vi "Add Device.vi"(8 "error in":errorcluster) -> (0 "error out":errorcluster)   [LabVIEW 2024, in "Data Base.lvlib"]
uses:
  Data Base.lvlib
  Support/General Type Defs/Global Data.vi
  Support/General Type Defs/General Type Defs.lvlib
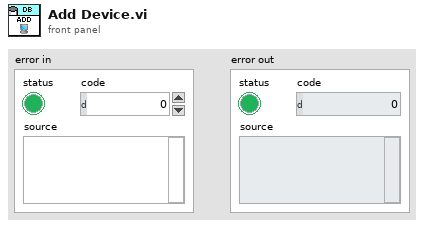
[diagram p1: front panel]
types:
  T1 = typedef "General Type Defs.lvlib/Device Data.ctl" = cluster{"OS":T2, "User":string, "Password":string, "Hostname":string, "IP Address":string}
  T2 = typedef "General Type Defs.lvlib/Device OS.ctl" = enum16{"Windows", "Linux"}
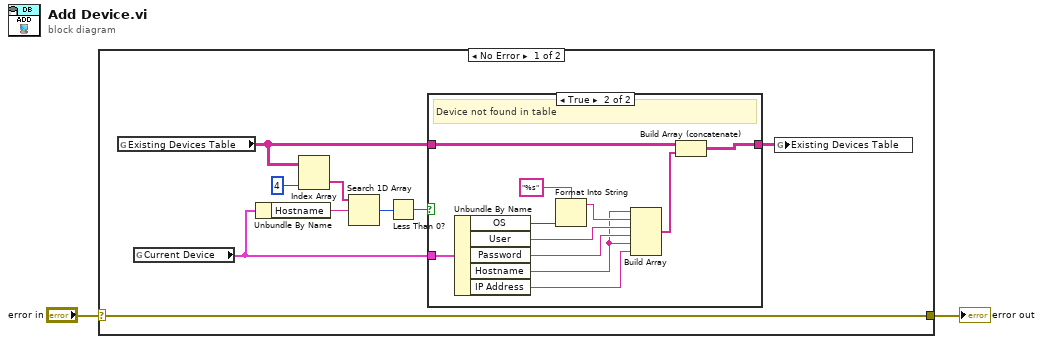
[diagram p0: block diagram]
diagram:
  n1 = case shown="No Error" "error in" {
    selector: "error in" -> [w5 w24]
    tunnel: [w5 w24] -> w1
    frame No Error {
      n2 = global read "Global Data.vi" "Existing Devices Table"() -> (w4:string[][])
      n3 = global read "Global Data.vi" "Current Device"() -> (w11:T1)
      n4 = Unbundle By Name(w11) -> ("Hostname"=w8:string)
      n5 = Index Array(array=w4, index (col)=4) -> (element=w9:string[])  [unwired: 1 in]
      n6 = Search 1D Array(1D array=w9, element=w8) -> (index of element=w7:i32)  [unwired: 1 in]
      n7 = Less Than 0?(x=w7) -> (x < 0?=w6:bool)
      n8 = case shown="True" w6 {
        tunnel: w11 -> [_ w23]
        tunnel: w4 -> [w12 w15]
        tunnel: [w12 w13] -> w3
        frame False {
          # "existing device in table"
        }
        frame True {
          # "Device not found in table"
          n9 = Unbundle By Name(w23) -> ("OS"=w22:T2, "User"=w19:string, "Password"=w18:string, "Hostname"=w16:string, "IP Address"=w17:string)
          n10 = Format Into String(format string="%s", w22) -> (resulting string=w20:string)  [unwired: 2 in, 1 out]
          n11 = Build Array(w16, w20, w19, w18, w16, w17) -> (w14:string[])
          n12 = Build Array (concatenate)(w15, w14) -> (w13:string[][])
        }
      }
      n13 = global write "Global Data.vi" "Existing Devices Table"(w3) -> ()
    }
    frame Error {
    }
  }
  "error out" <- w1
